vi "CaseStructures{6th}.vi"() -> ()   [LabVIEW 2023]
panel:
  in  "Numeric":dbl
  in  "STOP":bool
  out "Thermometer":dbl(slide) scale=0.0..150.0
  in  "temp":dbl(slide) scale=0.0..200.0
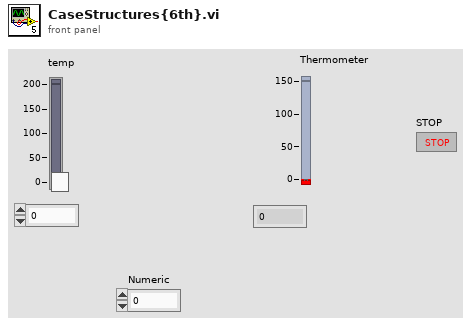
[diagram p1: front panel]
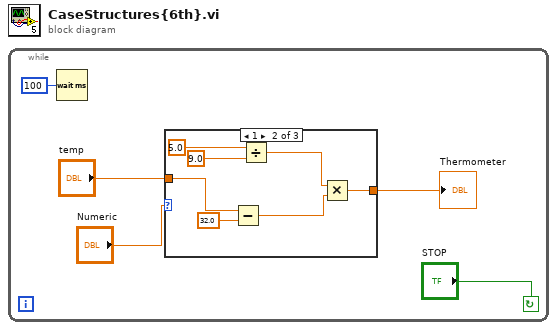
[diagram p0: block diagram]
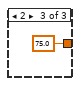
[diagram p3: hidden frame]
diagram:
  n1 = while {
    stop <- "STOP" continue-if-true
    n2 = Wait (ms)(milliseconds to wait=u32 100) -> ()  [unwired: 1 out]
    n3 = case shown="1" "Numeric" {
      tunnel: "temp" -> [w6 w10 _]
      tunnel: [w6 w7 75.0 ("temp")] -> w4
      frame 0, Default {
      }
      frame 1 {
        n4 = Subtract(x=w10, y=32.0) -> (x-y=w9:dbl)
        n5 = Divide(x=5.0, y=9.0) -> (x/y=w8:dbl)
        n6 = Multiply(x=w8, y=w9) -> (x*y=w7:dbl)
      }
      frame 2 {
      }
    }
    "Thermometer" <- w4
  }
